vi "Historical Table UI.vi"(8 "Reset Table Data":bool, 9 "Row Headers":string[](array[string]), 10 "Column Headers":string[](array[string]), 11 "Table Data":string[][](array[string])) -> ()   [LabVIEW 2024, in "Historical Table.lvlib" / "Historical Table.lvclass"]
uses:
  Historical Table.lvclass
panel:
  in  "Show Timestamps":bool
  in  "Pause Updating":bool
  out "Historical Data":string[][](table)
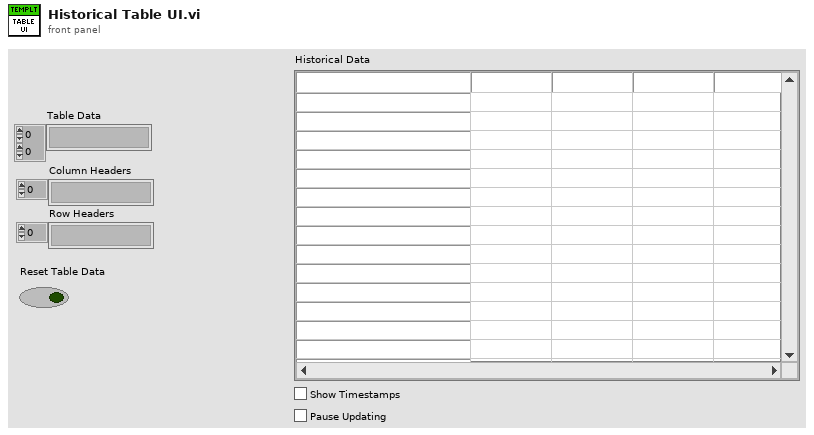
[diagram p1: front panel]
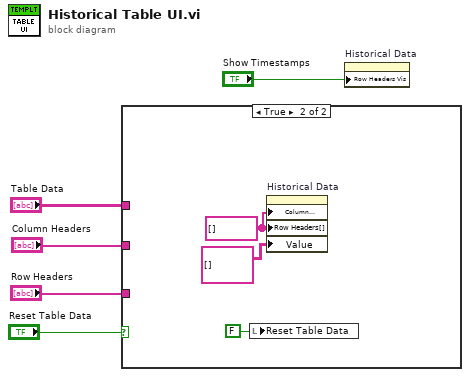
[diagram p0: block diagram]
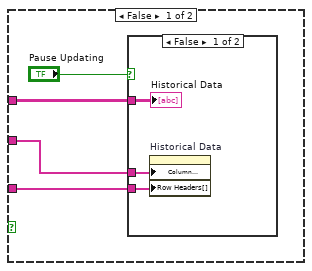
[diagram p2: hidden frame]
diagram:
  n1 = case shown="True" "Reset Table Data" {
    tunnel: "Table Data" -> [w7 _]
    tunnel: "Column Headers" -> [w9 _]
    tunnel: "Row Headers" -> [w8 _]
    frame False {
      n2 = case shown="False" "Pause Updating" {
        tunnel: w9 -> [w12 _]
        tunnel: w8 -> [w11 _]
        tunnel: w7 -> [w10 _]
        frame False {
          n3 = property on="Historical Data" class="Tbl (strict)"("Column Headers[]"=w12, "Row Headers[]"=w11) -> ()  [unwired: 2 in, 2 out]
          "Historical Data" <- w10
        }
        frame True {
        }
      }
    }
    frame True {
      w15 = string[] [] ("Row Header Strings[]")
      n4 = local write "Reset Table Data"(FALSE ("Reset Table Data")) -> ()
      n5 = property on="Historical Data" class="Tbl (strict)"("Column Headers[]"=w15, "Row Headers[]"=w15, "Value"=string[][] [] ("Historical Data")) -> ()  [unwired: 2 in, 2 out]
    }
  }
  n6 = property on="Historical Data" class="Tbl (strict)"("Row Headers Vis"="Show Timestamps") -> ()  [unwired: 2 in, 2 out]
